vi "Handle Error.vi"(8 "error in (no error)":errorcluster, 11 "IObserver in":refnum<class "IObserver.lvclass">) -> (0 "error out":errorcluster, 2 "stop actor?":bool=TRUE, 3 "IObserver out":refnum<class "IObserver.lvclass">)   [LabVIEW 2017, in "IObserver.lvlib" / "IObserver.lvclass"]
doc: "(<B>Filename</B>: Actor Framework.lvlib:Actor.lvclass:Handle Error.vi)\n\nDefines how the actor handles an error that occurred while processing a message. By default, this method does nothing except stop the actor."
uses:
  IObserver.lvclass
  <vilib>/ActorFramework/Actor/Actor.lvclass
  gpm_packages/@cs/event-logger/Source/Composed Log/Types/Log Level.ctl
  gpm_packages/@cs/event-logger/Source/Composed Log/Composed Log.lvlib
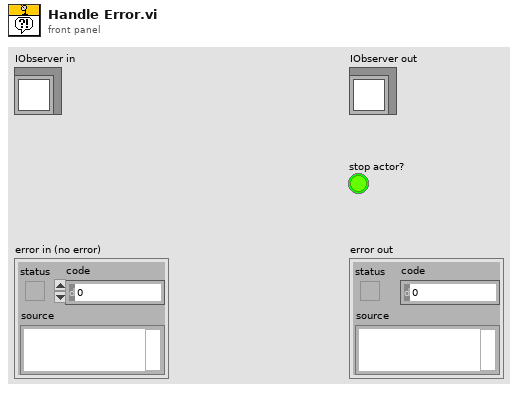
[diagram p1: front panel]
types:
  T1 = typedef "Composed Log.lvlib/Log Level.ctl" = enum16{"Debug", "Info", "Warning", "Error", "Critical"}
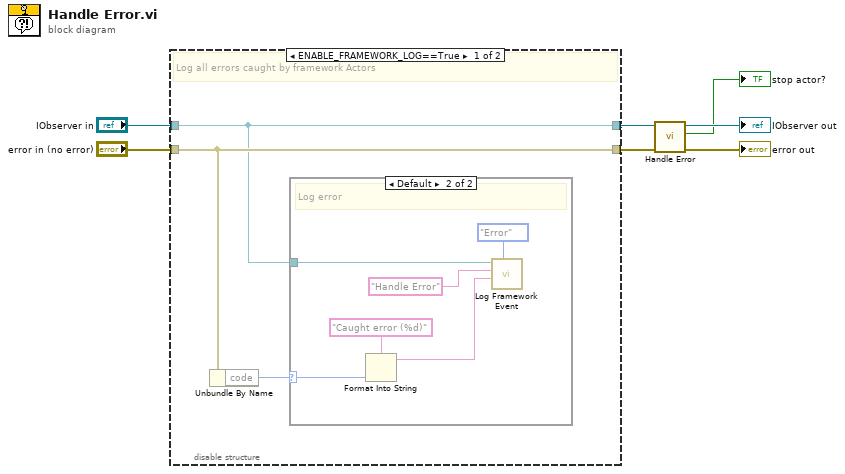
[diagram p0: block diagram]
diagram:
  n1 = disable-structure shown="ENABLE_FRAMEWORK_LOG==True" {
    disable-tunnel: "IObserver in" -> [w8 w18]
    disable-tunnel: [w8 w18] -> w2
    disable-tunnel: "error in (no error)" -> [w10 w17]
    disable-tunnel: [w10 w17] -> w1
    frame condition #0 {
      # "Log all errors caught by framework Actors"
      n2 = Unbundle By Name(w10) -> ("code"=w9:i32)
      n3 = case shown="Default" w9 {
        selector: w9 -> [_ w15]
        tunnel: w8 -> [_ w14]
        frame 43 {
          # "Normal shutdown -- Do not log"
        }
        frame Default {
          # "Log error"
          n4 = Format Into String(format string="Caught error (%d)", w15) -> (resulting string=w12:string)  [unwired: 2 in, 1 out]
          n5 = call "Log Framework Event.vi"("Event Level (Debug)"=Log_Level."Error", "Data To Log"=w12, "Caller Info (\"\")"="Handle Error" ("Caller Info (\"\")"), "IObserver in"=w14) -> ()  [unwired: 7 in, 1 out]
        }
      }
    }
    frame condition #1 (active) {
      # "Remove all logging from this method at compile time"
    }
  }
  n6 = call-parent "Handle Error.vi"("error in (no error)"=w1, "Actor in"=w2) -> ("error out"=→"error out":errorcluster, "stop actor?"=→"stop actor?":bool, "Actor out"=→"IObserver out":refnum<class "IObserver.lvclass">)  [unwired: 7 in]
